vi "Filter_test.vi"(7 "Headers":string[](array[string])=["Packet Number", "Timestamp", "Source", "Destination", "Protocol", "Length", "Data"], 10 "Filter String":string="Protocol == UDP AND Length > 0.7 OR Source == 192.168.1.1", 11 "Preiltered Data":string[][](array[string])=array1500x7[10500 elements]) -> (3 "Filtered Array":string[][](array[string]))   [LabVIEW 2025, in "Automotive Ethernet Bus Monitor UI.lvlib" / "Table_Filtering.lvlib"]
uses:
  Table_Filtering.lvlib
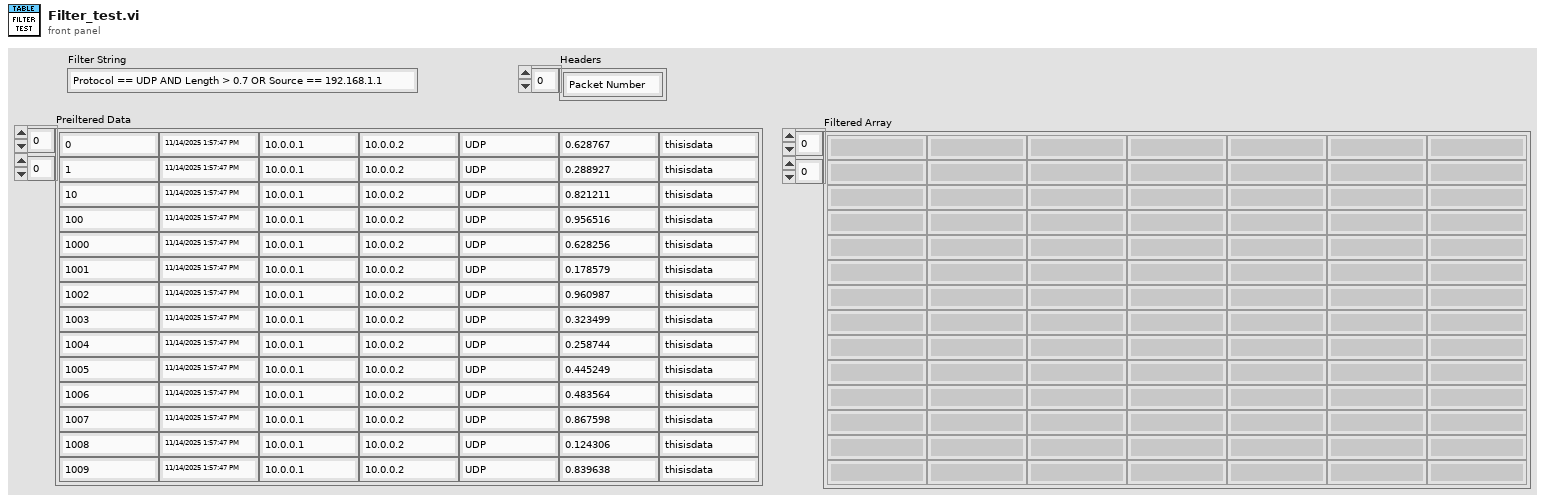
[diagram p1: front panel]
types:
  T1 = cluster{"FIELD":string, "OPERATOR":string, "VALUE":string}[]
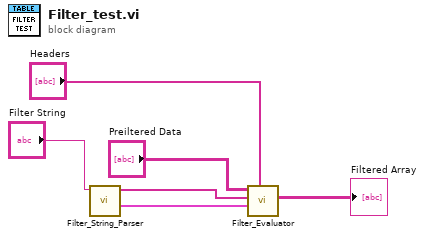
[diagram p0: block diagram]
diagram:
  n1 = call "Filter_String_Parser.vi"("Filter String"="Filter String") -> ("Comparators"=w5:T1, "Boolean Connectors"=w4:string[])  [unwired: 9 in]
  n2 = call "Filter_Evaluator.vi"("Headers"="Headers", "Comparators"=w5, "Boolean Connectors"=w4, "Prefiltered Data"="Preiltered Data") -> ("Filtered Array"=→"Filtered Array":string[][])  [unwired: 6 in, 1 out]
